vi "Pulse generator.vi"() -> ()   [LabVIEW 2013]
panel:
  in  "Stop":bool
  in  "Repetition":i32=50
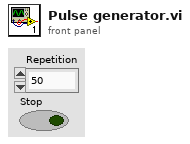
[diagram p1: front panel]
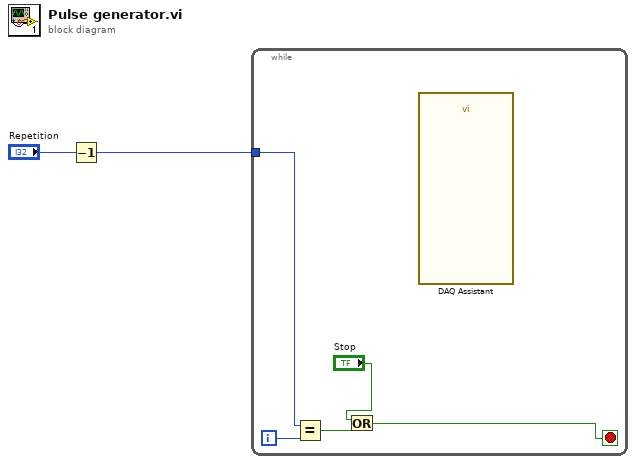
[diagram p0: block diagram]
diagram:
  n1 = Decrement(x="Repetition") -> (x-1=w1:i32)
  n2 = while {
    tunnel: w1 -> [w6]
    i -> [w7]
    stop <- w3 stop-if-true
    n3 = Equal?(x=w6, y=w7) -> (x = y?=w5:bool)
    n4 = Or(x="Stop", y=w5) -> (x .or. y?=w3:bool)
    n5 = call "DAQ Assistant"() -> ()  [unwired: 18 in, 2 out]
  }
